vi "AutoSetClaw.vi"(8 "error in (no error)":errorcluster, 11 "ClawDemand":dbl) -> (0 "error out":errorcluster)   [LabVIEW 2023]
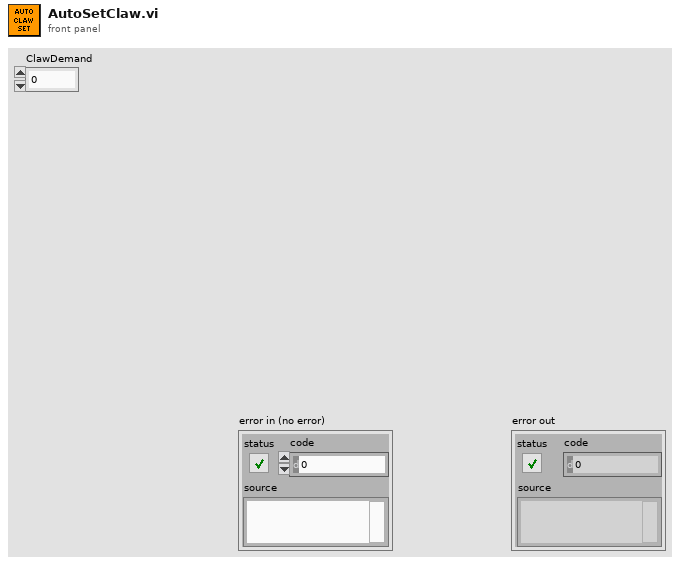
[diagram p1: front panel]
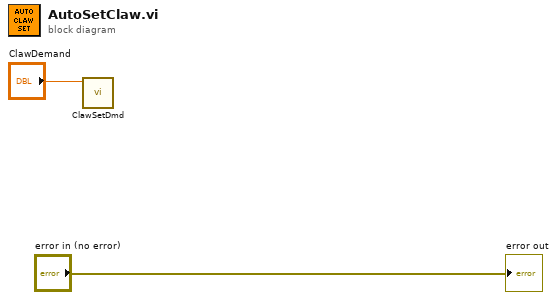
[diagram p0: block diagram]
diagram:
  n1 = call "ClawSetDmd.vi"("ClawDemand"="ClawDemand") -> ()  [unwired: 11 in]
  "error out" <- "error in (no error)"
